vi "PC_CallRTGuidedMunitions.vi"(4 "Value":variant, 6 "Control Name":string="InputControl", 7 "Machine":string="192.168.120.8", 8 "error in (no error)":errorcluster, 9 "SetControl?":bool, 10 "Reentrant?":bool, 11 "VIPath":path=path "C:/ni-rt/startup/Test.vi") -> (0 "error out":errorcluster, 3 "Control Value:Get All":cluster{"Name":string, "Variant Data":variant}[](array[cluster]))   [LabVIEW 2010]
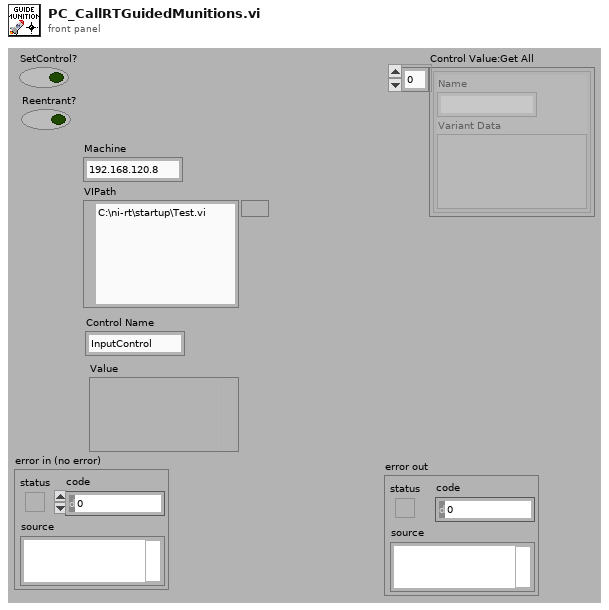
[diagram p1: front panel]
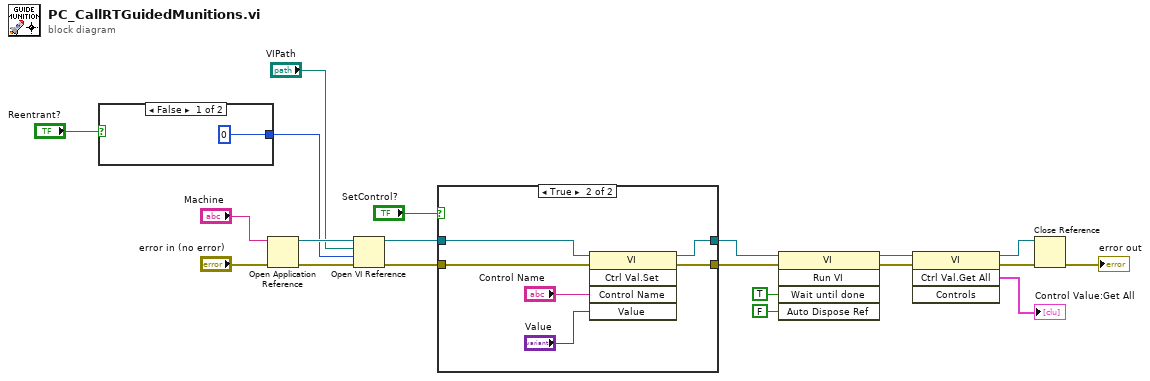
[diagram p0: block diagram]
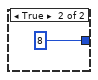
[diagram p2: hidden frame]
diagram:
  n1 = case shown="False" "Reentrant?" {
    tunnel: [0 ("options") 8 ("options")] -> w14
    frame False {
    }
    frame True {
    }
  }
  n2 = Open Application Reference(8:"error in (no error)", 11:"Machine") -> (0:w18:errorcluster, 3:w19:refnum<vi>)  [unwired: 2 in]
  n3 = Open VI Reference(application reference (local)=w19, vi path="VIPath", options=w14, error in (no error)=w18) -> (vi reference=w13:refnum<vi>, error out=w11:errorcluster)  [unwired: 2 in]
  n4 = case shown="True" "SetControl?" {
    tunnel: w13 -> [w23 w29]
    tunnel: [w23 w28] -> w12
    tunnel: w11 -> [w24 w27]
    tunnel: [w24 w26] -> w10
    frame False {
    }
    frame True {
      n5 = invoke class="VI" method="Ctrl Val.Set"(reference=w29, error in=w27, "Control Name"="Control Name", "Value"="Value") -> (reference out=w28:refnum<vi>, error out=w26:errorcluster)  [unwired: 1 in, 3 out]
    }
  }
  n6 = invoke class="VI" method="Run VI"(reference=w12, error in=w10, "Wait until done"=TRUE ("Wait Until Done"), "Auto Dispose Ref"=FALSE ("Auto Dispose Reference")) -> (reference out=w6:refnum<vi>, error out=w5:errorcluster)  [unwired: 1 in, 3 out]
  n7 = invoke class="VI" method="Ctrl Val.Get All"(reference=w6, error in=w5) -> (reference out=w3:refnum<vi>, error out=w4:errorcluster, "Get All Control Values Variant"=→"Control Value:Get All":cluster{"Name":string, "Variant Data":variant}[])  [unwired: 2 in, 1 out]
  n8 = Close Reference(reference=w3, error in (no error)=w4) -> (error out=→"error out":errorcluster)
